vi "ramping Output.vi"(10 "Speed":dbl, 11 "Max Change":dbl) -> (3 "New Speed":dbl)   [LabVIEW 2014]
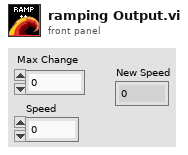
[diagram p1: front panel]
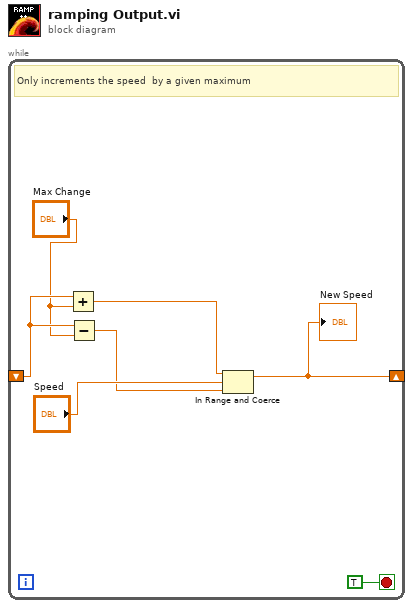
[diagram p0: block diagram]
diagram:
  n1 = while {
    shift-right: [w6] -> _
    shift-left: _ -> [w3]
    stop <- TRUE stop-if-true
    # "Only increments the speed  by a given maximum"
    n2 = Add(x=w3, y="Max Change") -> (x+y=w5:dbl)
    n3 = Subtract(x=w3, y="Max Change") -> (x-y=w4:dbl)
    n4 = In Range and Coerce(upper limit=w5, x="Speed", lower limit=w4) -> (coerced(x)=w6:dbl)  [unwired: 1 out]
    "New Speed" <- w6
  }
